vi "SetTorqueAndSpeed.vi"(8 "error in (no error)":errorcluster, 9 "Speed":i32, 10 "Torque":sgl, 11 "Cluster in":T1) -> (0 "error out":errorcluster, 3 "Cluster out":T1)   [LabVIEW 2019]
uses:
  core_dataRefCluster.ctl
  core_dataRef.ctl
  core_dataCluster.ctl
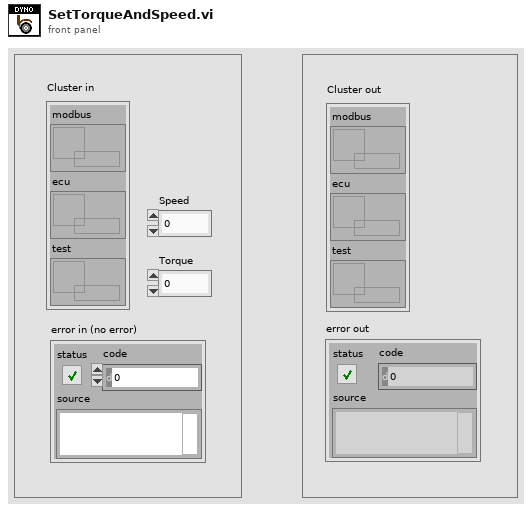
[diagram p1: front panel]
types:
  T1 = typedef "core_dataRefCluster.ctl" = cluster{"modbus":T2, "ecu":T2, "test":T2}
  T2 = typedef "core_dataRef.ctl" = refnum<queue>
  T3 = typedef "core_dataCluster.ctl" = cluster{"cmd":string, "data":variant}
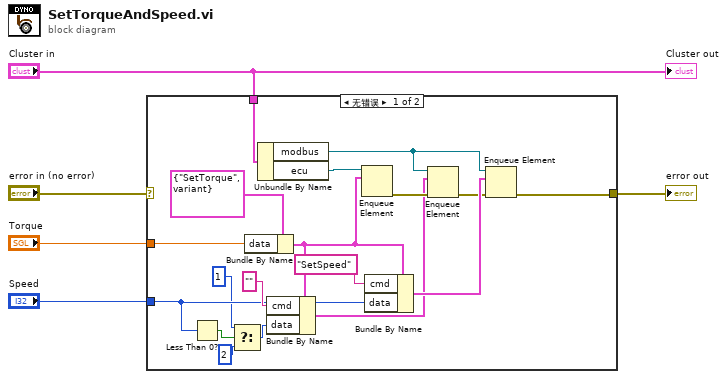
[diagram p0: block diagram]
diagram:
  n1 = case shown="无错误" "error in (no error)" {
    selector: "error in (no error)" -> [_ w24]
    tunnel: "Torque" -> [w21 _]
    tunnel: "Cluster in" -> [w20 _]
    tunnel: [w19 w24] -> w3
    tunnel: "Speed" -> [w10 _]
    frame No Error {
      n2 = Less Than 0?(x=w10) -> (x < 0?=w8:bool)
      n3 = Select(t=1, s=w8, f=2) -> (s? t:f=w9:i32)
      n4 = Bundle By Name(cluster=T3 {"cmd"="SetTorque", "data"=variant} ("element"), "data"=w21) -> (w12:T3)
      n5 = Unbundle By Name(w20) -> ("modbus"=w16:T2, "ecu"=w23:T2)
      n6 = Bundle By Name(cluster=w12, "cmd"="", "data"=w9) -> (w13:T3)
      n7 = Enqueue Element(queue=w23, element=w12) -> (error out=w15:errorcluster)  [unwired: 2 in, 2 out]
      n8 = Bundle By Name(cluster=w12, "cmd"="SetSpeed", "data"=w10) -> (w18:T3)
      n9 = Enqueue Element(queue=w16, element=w13, error in (no error)=w15) -> (error out=w14:errorcluster)  [unwired: 1 in, 2 out]
      n10 = Enqueue Element(queue=w16, element=w18, error in (no error)=w14) -> (error out=w19:errorcluster)  [unwired: 1 in, 2 out]
    }
    frame Error {
    }
  }
  "error out" <- w3
  "Cluster out" <- "Cluster in"
